vi "Catch Multiple Exceptions.vi"(0 "targets":refnum<class "Exception.lvclass">[](array[class]), 11 "error in (no error)":errorcluster) -> (4 "catched exception":refnum<class "Exception.lvclass">, 6 "catched":bool, 15 "error out":errorcluster)   [LabVIEW 2015, in "LV Exceptions v1.lvlib"]
doc: "Catches the exception: error cluster that contains exception is cleared and exception is extracted as an object. Only exceptions of target class or descending classes are catched.\n\nMultiple target classes can be specified.\n\nError cluster which doesn't contain exception will not be cleared.\n\nIf error cluster contains exception, but it cannot be extracted successfully, this functions returns error that describes the reason. Original Exception is overwritten."
uses:
  LV Exceptions v1.lvlib
  Exception/Exception.lvclass
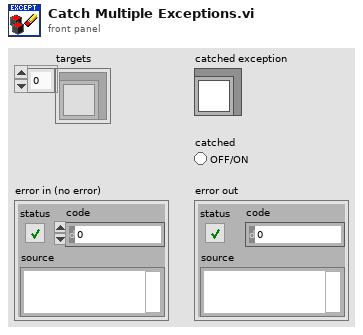
[diagram p1: front panel]
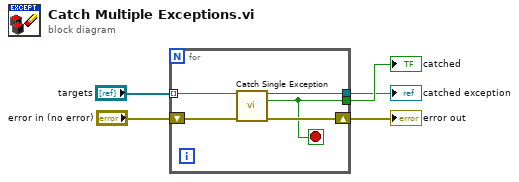
[diagram p0: block diagram]
diagram:
  n1 = for {
    shift-right: [w8] -> w2
    shift-left: "error in (no error)" -> [w10]
    tunnel: "targets" -> [w9] mode=indexing
    tunnel: [w7] -> w4
    tunnel: [w6] -> w5
    stop <- w6 stop-if-true
    n2 = call "Catch Single Exception.vi"("target"=w9, "error in (no error)"=w10) -> ("catched exception out"=w7:refnum<class "Exception.lvclass">, "catched"=w6:bool, "error out"=w8:errorcluster)  [unwired: 11 in]
  }
  "catched" <- w5
  "catched exception" <- w4
  "error out" <- w2
